vi "Lab 9 Exercise 7 - Square Root.vi"() -> ()   [LabVIEW 2023]
panel:
  out "error out":errorcluster
  in  "error in (no error)":errorcluster
  out "Square Root":dbl
  in  "Square Root Input":dbl
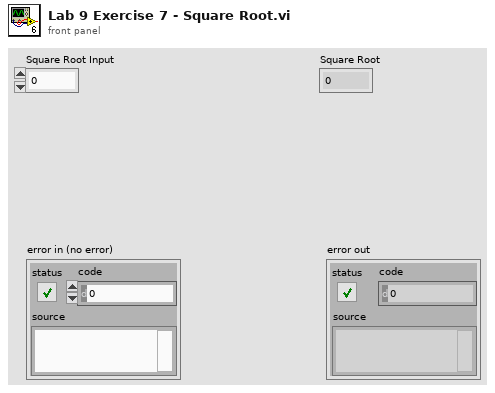
[diagram p1: front panel]
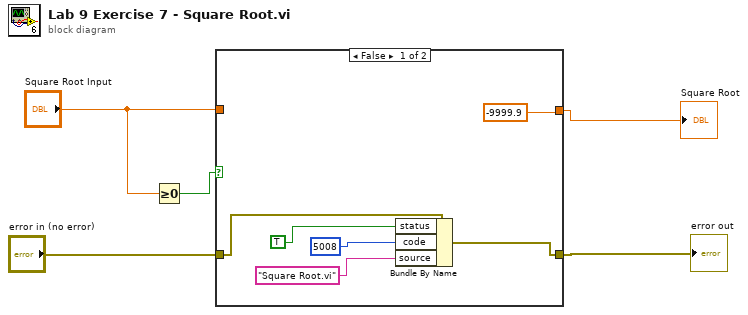
[diagram p0: block diagram]
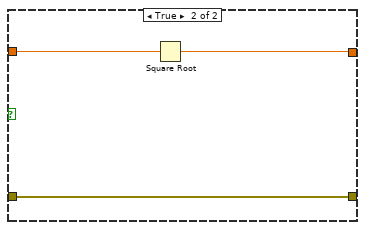
[diagram p2: hidden frame]
diagram:
  n1 = Greater Or Equal To 0?(x="Square Root Input") -> (x >= 0?=w3:bool)
  n2 = case shown="False" w3 {
    tunnel: "Square Root Input" -> [_ w14]
    tunnel: [-9999.9 w13] -> w5
    tunnel: "error in (no error)" -> [w10 w12]
    tunnel: [w9 w12] -> w1
    frame False {
      n3 = Bundle By Name(cluster=w10, "status"=TRUE, "code"=5008, "source"="Square Root.vi") -> (w9:errorcluster)
    }
    frame True {
      n4 = Square Root(x=w14) -> (sqrt(x)=w13:dbl)
    }
  }
  "Square Root" <- w5
  "error out" <- w1
